vi "PH_SHS_Analysis_Calibrator.calibration data file.vi"(0 "Camera Instance":string="DummyCam", 1 "Method":enum16{"automatic", "manual"}(ring), 2 "Time of Calibration Data saving":timestamp, 5 "error in":errorcluster) -> (11 "File extension":string=".dat", 13 "Methods":string[](array[string])=["Auto", "Man"], 14 "File to save SHS Analysis Calibration Data in":path, 15 "Directory path to save  SHS Analysis Calibration Data in":path=path "D:/PCS/SHS", 16 "Deliminator":string="---", 17 "Type of Data":string="SHS_Anal_Cali", 18 "Structure of File Name":string, 19 "error out":errorcluster)   [LabVIEW 2014, in "PH_SHS_Analysis_Calibrator.lvlib"]
doc: "This VI is forseen to be used in the save data file VI as well as in VIs used to read data from hard disk. If all inputs are connected, this VI creates a file name; at the outputs, you can check the result: \"Type of Data\" is the starting part of the name and so on. \"Structure of File Name\" explains the components for further use."
uses:
  PH_SHS_Analysis_Calibrator.lvlib
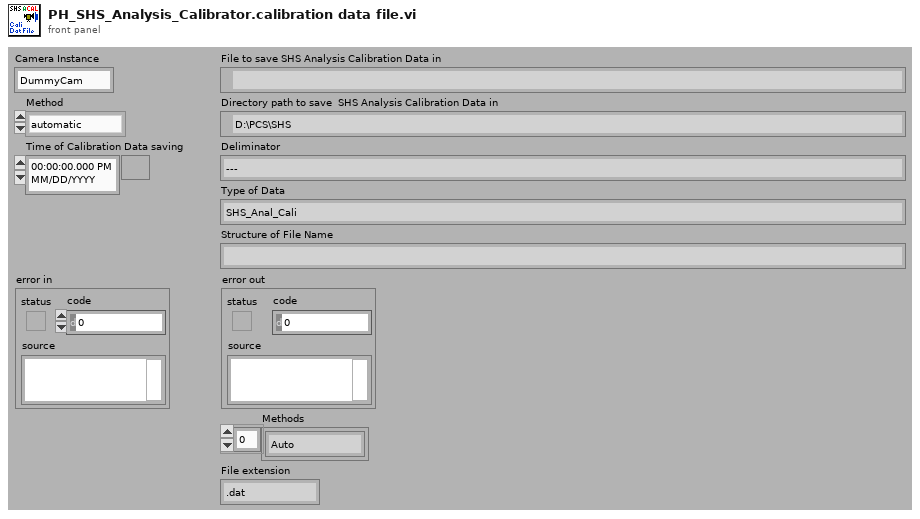
[diagram p1: front panel]
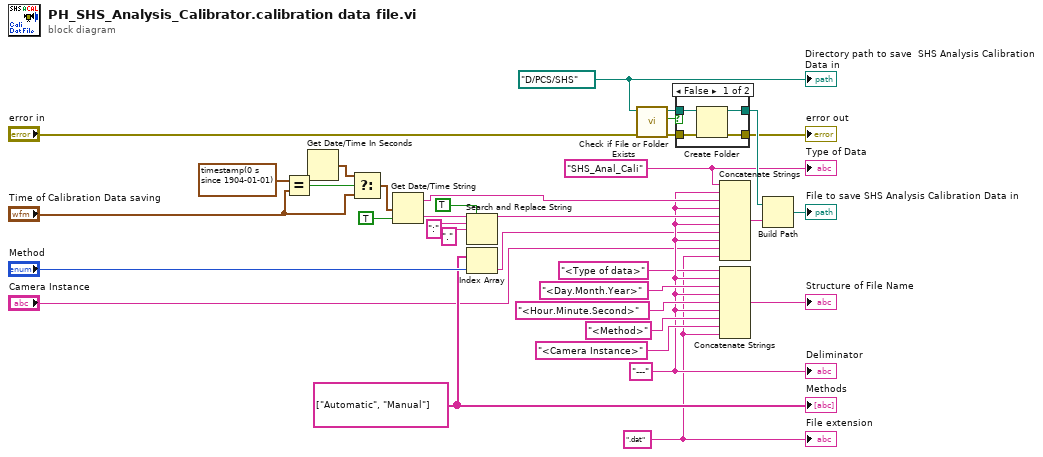
[diagram p0: block diagram]
diagram:
  w25 = path "D:/PCS/SHS" ("base path")
  w5 = string[] ["Automatic", "Manual"]
  w23 = "SHS_Anal_Cali" ("string")
  w9 = "---"
  w2 = ".dat" ("string")
  n1 = Equal?(x=timestamp(0 s since 1904-01-01) ("y"), y="Time of Calibration Data saving") -> (x = y?=w18:bool)
  n2 = Get Date/Time In Seconds() -> (seconds since 1Jan1904=w14:timestamp)
  n3 = Select(t=w14, s=w18, f="Time of Calibration Data saving") -> (s? t:f=w15:timestamp)
  n4 = Get Date/Time String(seconds (now)=w15, want seconds? (F)=TRUE) -> (date string=w34:string, time string=w32:string)  [unwired: 1 in]
  n5 = Search and Replace String(replace all?=TRUE ("replace all? (F)"), input string=w32, search string=":", replace string="." ("replace string (\"\")")) -> (result string=w19:string)  [unwired: 4 in, 3 out]
  n6 = Index Array(array=w5, index="Method") -> (element=w4:string)
  n7 = call <vilib>:"Check if File or Folder Exists.vi"("error in (no error)"="error in", "path"=w25) -> ("error out"=w27:errorcluster, "file or folder exists?"=w26:bool, "dup path"=w28:path)  [unwired: 7 in]
  n8 = case shown="False" w26 {
    tunnel: w27 -> [w37 w39]
    tunnel: w28 -> [w38 w40]
    tunnel: [w35 w40] -> w31
    tunnel: [w36 w39] -> w29
    frame False {
      n9 = Create Folder(path (use dialog)=w38, error in=w37) -> (created path=w35:path, error out=w36:errorcluster)  [unwired: 1 in, 1 out]
    }
    frame True {
    }
  }
  "error out" <- w29
  n10 = Concatenate Strings(w23, w9, w34, w9, w19, w9, w4, w9, "Camera Instance", w2) -> (w24:string)
  n11 = Concatenate Strings("<Type of data>" ("string"), w9, "<Day.Month.Year>" ("string"), w9, "<Hour.Minute.Second>" ("string"), w9, "<Method>" ("string"), "<Camera Instance>" ("string"), w2) -> (→"Structure of File Name":string)
  n12 = Build Path(base path=w31, name or relative path=w24) -> (appended path=→"File to save SHS Analysis Calibration Data in":path)
  "Directory path to save  SHS Analysis Calibration Data in" <- w25
  "Deliminator" <- w9
  "Type of Data" <- w23
  "Methods" <- w5
  "File extension" <- w2
